vi "Post-Run.vi"(8 "error in":errorcluster, 11 "Actor in":refnum<class "Actor.lvclass">) -> (0 "error out":errorcluster, 3 "Actor out":refnum<class "Actor.lvclass">)   [LabVIEW 2018, in "Actor.lvclass"]
uses:
  Actor.lvclass
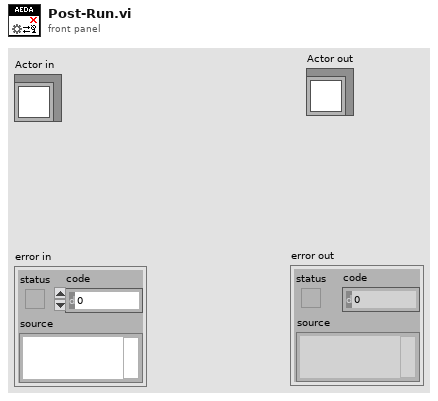
[diagram p1: front panel]
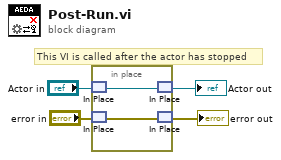
[diagram p0: block diagram]
diagram:
  # "This VI is called after the actor has stopped"
  n1 = in-place {
    n2 = in-place-match #1("Actor in") -> (w5:refnum<class "Actor.lvclass">)
    n3 = in-place-match #2("error in") -> (w6:errorcluster)
    n4 = in-place-match #1(w5) -> (→"Actor out":refnum<class "Actor.lvclass">)
    n5 = in-place-match #2(w6) -> (→"error out":errorcluster)
  }
